vi "Read From TCP.vi"(5 "Upload Path (Temp)":path=path "", 6 "Max Size (50MB)":u64=52428800, 7 "Uploads as Files? (T)":bool=TRUE, 8 "error in (no error)":errorcluster, 9 "TCP Connection":refnum<k5>, 10 "Client URI":refnum<class "URI.lvclass">) -> (0 "error out":errorcluster, 3 "Request out":refnum<class "Request.lvclass">)   [LabVIEW 2020, in "HTTP Utils.lvlib" / "Request.lvclass"]
uses:
  Request.lvclass
  lv-uri/URI/URI/URI.lvclass
  Request.lvclass/Request.ctl
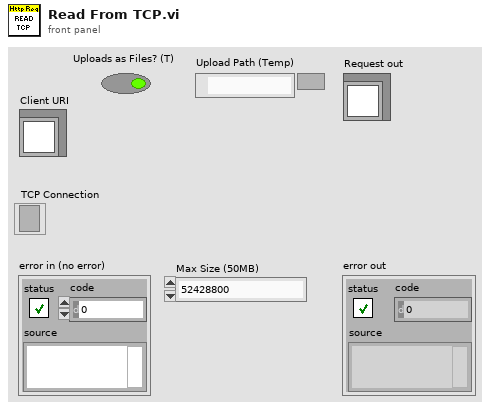
[diagram p1: front panel]
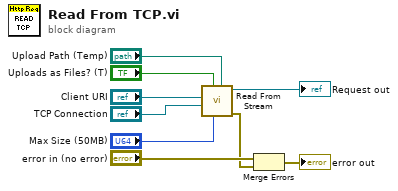
[diagram p0: block diagram]
diagram:
  n1 = call "Read From Stream.vi"("Upload Path (Temp)"="Upload Path (Temp)", "Max Size (50MB)"="Max Size (50MB)", "Uploads as Files? (T)"="Uploads as Files? (T)", "TCP in"="TCP Connection", "Client URI"="Client URI") -> ("error out"=w6:errorcluster, "Request out"=→"Request out":refnum<class "Request.lvclass">)  [unwired: 4 in, 1 out]
  n2 = Merge Errors("error in (no error)", w6) -> (→"error out":errorcluster)
